vi "toTimestamp.vi"(7 "Use TAI Offset?":bool, 9 "Fractional Second":dbl format="%#.6f", 10 "Unix Time (s)":i64, 11 "Epoch (Unix)":refnum<class "Epoch.UNIX.lvclass">) -> (1 "Not a Timestamp?":bool, 2 "Timestamp":timestamp, 3 "Epoch out":refnum<class "Epoch.UNIX.lvclass">)   [LabVIEW 2013, in "Epoch.UNIX.lvclass"]
uses:
  Epoch.UNIX.lvclass
  epoch/Epoch.lvclass
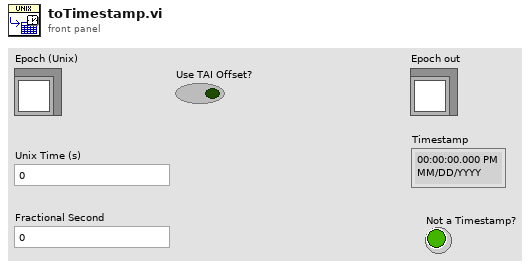
[diagram p1: front panel]
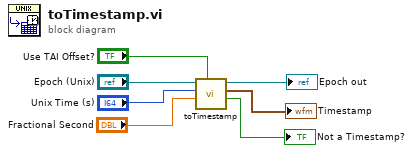
[diagram p0: block diagram]
diagram:
  n1 = call-parent "toTimestamp.vi"("Use TAI Offset?"="Use TAI Offset?", "Fractional Second"="Fractional Second", "Epoch Time (s)"="Unix Time (s)", "Epoch (Local)"="Epoch (Unix)") -> ("Not a Timestamp?"=→"Not a Timestamp?":bool, "Timestamp"=→"Timestamp":timestamp, "Epoch (out)"=→"Epoch out":refnum<class "Epoch.UNIX.lvclass">)  [unwired: 5 in]
